vi "lockin_simulated.vi"() -> ()   [LabVIEW 2015]
uses:
  <vilib>/express/express analysis/Spectral/Block/exnSpectralBlock spectral measurements power poly.vi
  <vilib>/express/express analysis/Spectral/Block/exnSpectralBlock spectral measurements power DDT.vi
  <vilib>/express/express analysis/Spectral/XNode/ExpressSpectralMeasurementsBlockNode.xnode
  <vilib>/Analysis/NI_AALPro.lvlib
panel:
  out "Final Output (filtered) (2f+dc)":dynamicdata(graph) caption="Sine"
  in  "stop":bool
  out "Noise":dynamicdata(graph) caption="Sine"
  out "Noise+Input":dynamicdata(graph) caption="Sine"
  in  "Phase":dbl(slide) scale=0.0..180.0
  out "Reference":dynamicdata(graph) caption="Sine"
  out "Demodulated Output 2":dbl(knob) scale=-0.35..0.35
  out "Final Output (2f+dc) 2":dynamicdata(graph) caption="Sine"
  out "AC estimate (Vrms)":dbl(knob) scale=0.0..1.0
  out "Filtered Signal":dynamicdata(graph)
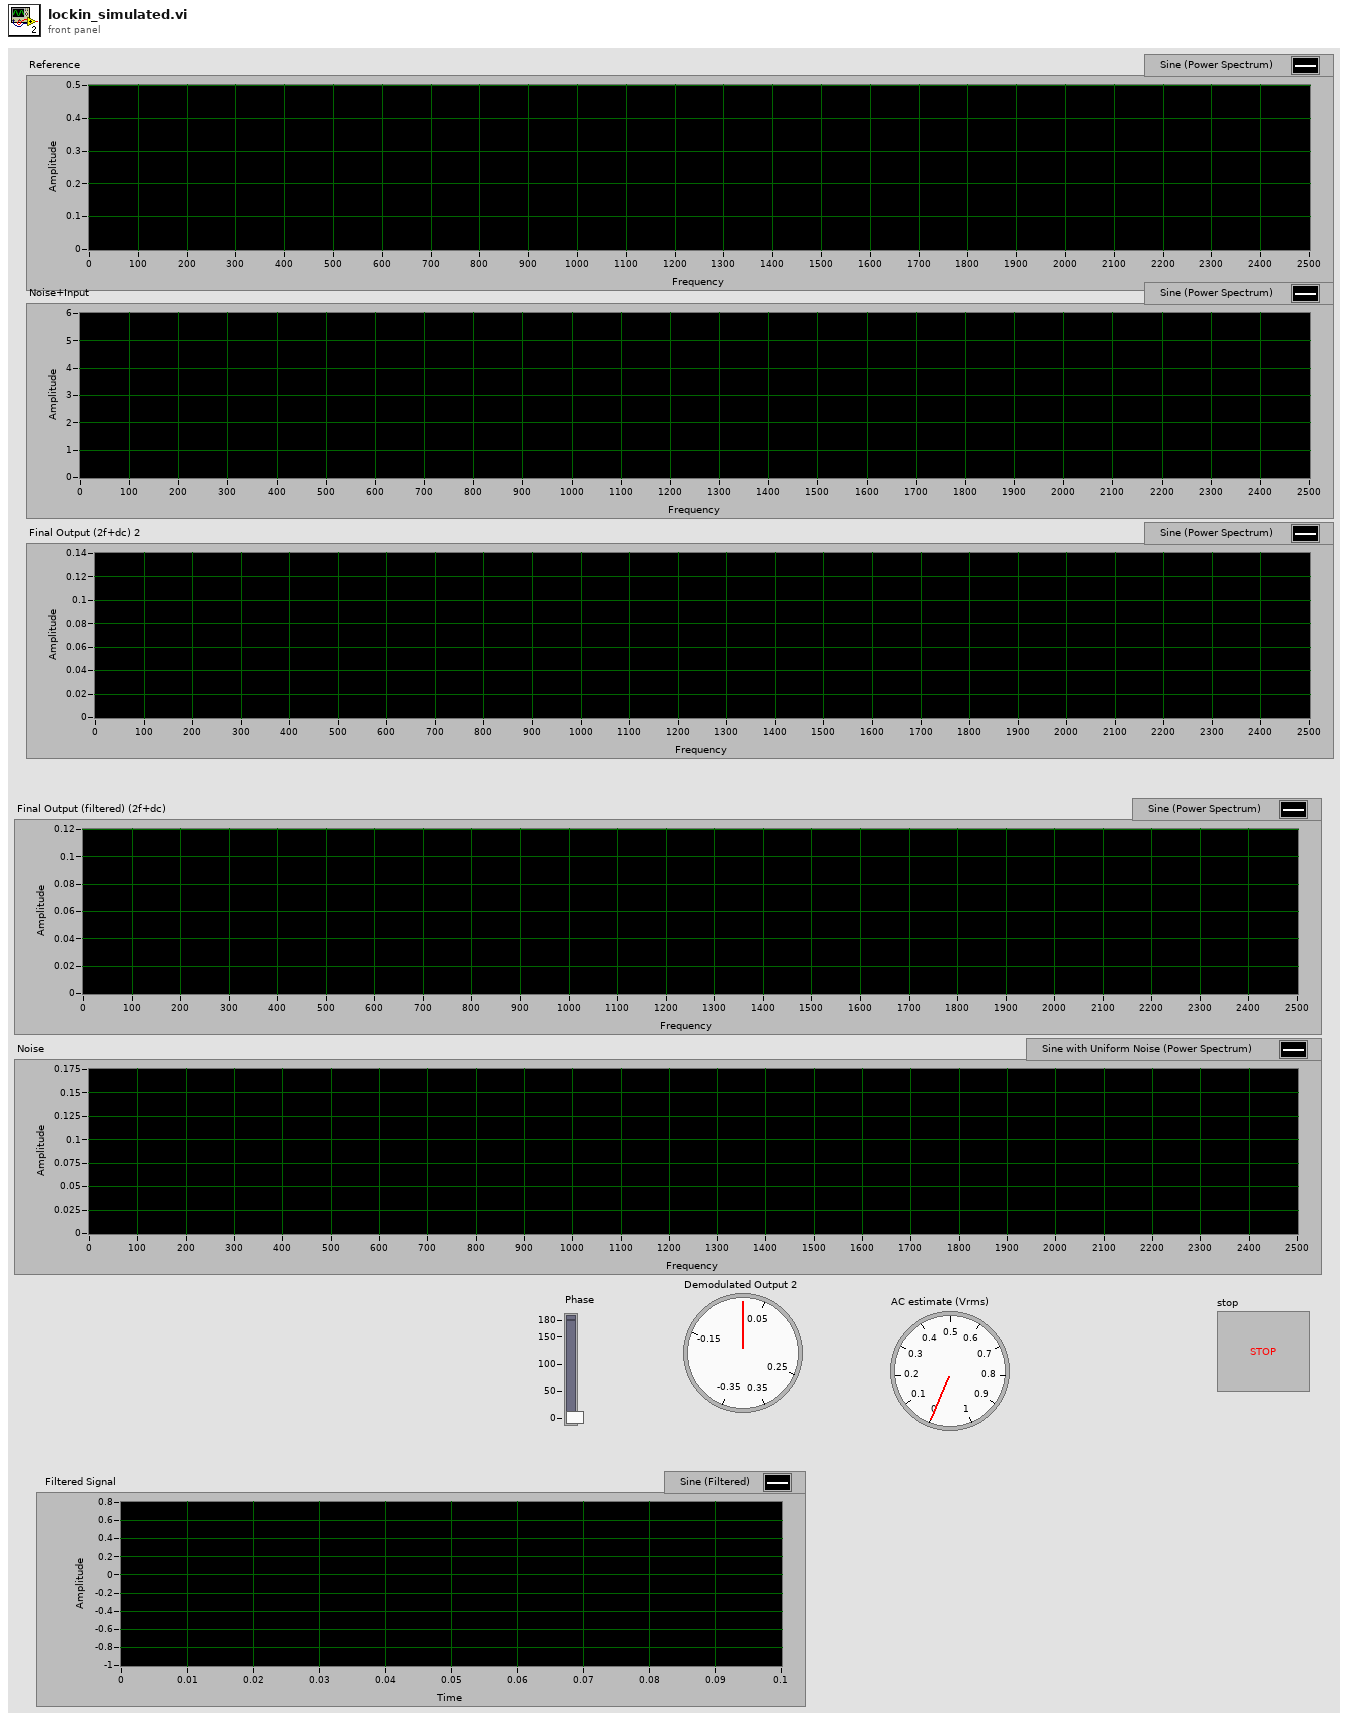
[diagram p1: front panel]
types:
  T1 = cluster{"averaging mode":u16, "weighting mode":u16, "number of averages":u32}
  T2 = cluster{"dB On (F)":bool, "unwrap phase (F)":bool, "convert to degree (F)":bool}
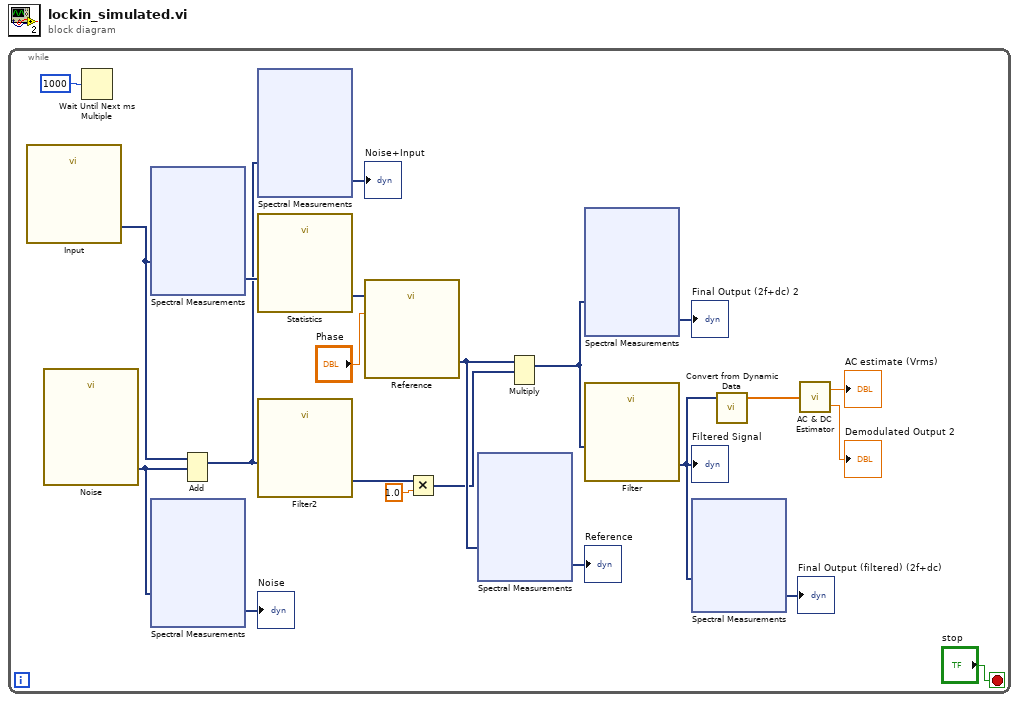
[diagram p0: block diagram]
diagram:
  n1 = while {
    stop <- "stop" stop-if-true
    n2 = call "Input"() -> ("Sine"=w21:dynamicdata)  [unwired: 14 in, 1 out]
    n3 = call "Noise"() -> ("Sine with Uniform Noise"=w4:dynamicdata)  [unwired: 14 in, 1 out]
    n4 = Wait Until Next ms Multiple(millisecond multiple=u32 1000) -> ()  [unwired: 1 out]
    n5 = xnode "Spectral Measurements"("Signals"=w21) -> ("Power Spectrum"=w19:dynamicdata)  [unwired: 1 in, 1 out]
    n6 = xnode "Spectral Measurements"("Signals"=w4) -> ("Power Spectrum"=→"Noise":dynamicdata)  [unwired: 1 in, 1 out]
    n7 = Add(1:w4, 2:w21) -> (0:w2:dynamicdata)  [unwired: 1 in, 1 out]
    n8 = xnode "Spectral Measurements"("Signals"=w2) -> ("Power Spectrum"=→"Noise+Input":dynamicdata)  [unwired: 1 in, 1 out]
    n9 = call "Statistics"("Signals"=w19) -> ("Time of Maximum"=w18:dynamicdata)  [unwired: 25 in, 1 out]
    n10 = call "Filter2"("Signal"=w2) -> ("Filtered Signal"=w1:dynamicdata)  [unwired: 9 in, 1 out]
    n11 = call "Reference"("Frequency"=w18, "Phase"="Phase") -> ("Sine"=w10:dynamicdata)  [unwired: 12 in, 1 out]
    n12 = Multiply(x=w1, y=1.0) -> (x*y=w7:dynamicdata)
    n13 = xnode "Spectral Measurements"("Signals"=w10) -> ("Power Spectrum"=→"Reference":dynamicdata)  [unwired: 1 in, 1 out]
    n14 = Multiply(1:w7, 2:w10) -> (0:w9:dynamicdata)  [unwired: 1 in, 1 out]
    n15 = xnode "Spectral Measurements"("Signals"=w9) -> ("Power Spectrum"=→"Final Output (2f+dc) 2":dynamicdata)  [unwired: 1 in, 1 out]
    n16 = call "Filter"("Signal"=w9) -> ("Filtered Signal"=w6:dynamicdata)  [unwired: 9 in, 1 out]
    "Filtered Signal" <- w6
    n17 = xnode "Spectral Measurements"("Signals"=w6) -> ("Power Spectrum"=→"Final Output (filtered) (2f+dc)":dynamicdata)  [unwired: 1 in, 1 out]
    n18 = call "Convert from Dynamic Data"("Dynamic Data Type"=w6) -> ("Array"=w8:dbl[])  [unwired: 3 in]
    n19 = call <vilib>:"AC & DC Estimator.vi"("Signal (V)"=w8) -> ("AC estimate (Vrms)"=→"AC estimate (Vrms)":dbl, "DC estimate (V)"=→"Demodulated Output 2":dbl)
  }
